vi "saturate.vi"(2 "amplitude":dbl, 3 "value":dbl) -> (0 "sat":bool, 1 "saturated":dbl)   [LabVIEW 2014]
uses:
  <vilib>/imath/engines/lvmath2/RunTimeEngine/NodeEndStatement/NIMS_NodeEndStatement_Output.vi
  <instcachedir>/0/NIMS_NodeEndStatement_Output_53EC0D466D134D7ABD903AC30B43404B.lvgen/NIMS_NodeEndStatement_Output_53EC0D466D134D7ABD903AC30B43404B_001.vi
  <instcachedir>/0/NIMS_NodeEndStatement_Output_53EC0D466D134D7ABD903AC30B43404B.lvgen/NIMS_NodeEndStatement_Output_53EC0D466D134D7ABD903AC30B43404B_011.vi
  <vilib>/imath/engines/lvmath2/RunTimeEngine/ErrorHandling/NIMS_Finalize Error.vi
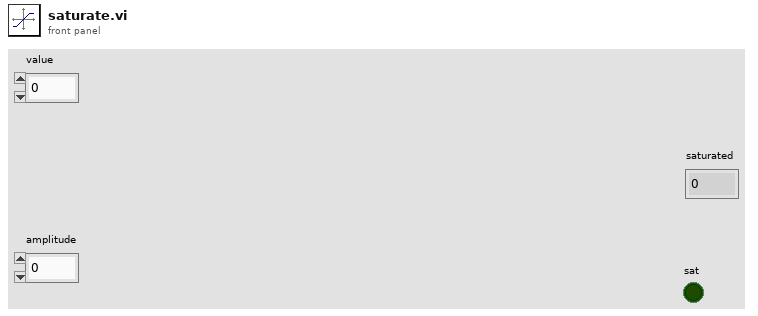
[diagram p1: front panel]
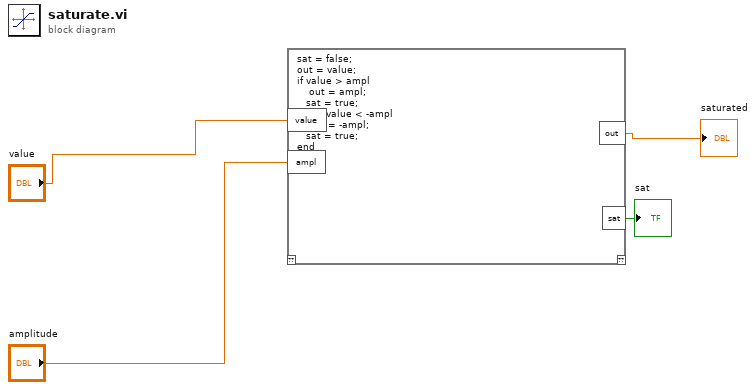
[diagram p0: block diagram]
diagram:
  n1 = mathscript code="sat = false;\nout = value;\nif value > ampl\n    out = ampl;\n   sat = true;\nelseif value < -ampl\n    out = -ampl;\n   sat = true;\nend"("value"="value", "ampl"="amplitude") -> ("out"=→"saturated":dbl, "sat"=→"sat":bool)  [unwired: 1 in, 1 out]
